vi "Get Editor .NET.vi"(11 "Editor Control Base in":refnum<class "Editor Control Base.lvclass">) -> (2 "Editor Control .NET":refnum<k24>, 3 "Editor Control Base out":refnum<class "Editor Control Base.lvclass">)   [LabVIEW 2023, in "SourceGrid.lvlib" / "Editor Control Base.lvclass"]
uses:
  Editor Control Base.lvclass
  D:/git/Sourcegrid-LabVIEW/dll/SourceGrid.dll
  dll/SourceGrid.dll
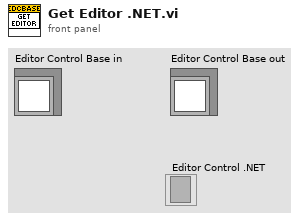
[diagram p1: front panel]
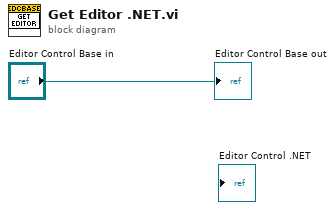
[diagram p0: block diagram]
diagram:
  "Editor Control Base out" <- "Editor Control Base in"
